vi "AudioTest.SoundCheck Data Log Graph Window - Composite_Smaller.vi"() -> ()   [LabVIEW 2018]
uses:
  TypeDefs/AudioTest.Analysis Data Record.ctl
  TypeDefs/AudioTest.Analysis Folder Navigation Status.ctl
  <vilib>/KATE/Queues/Queue Utils.lvlib
panel:
  in  "Main Tab":enum32{"Data", "Setup"}(tab)
  out "Cmnt":string
  out "Mic Covered Level":string caption="Covered"
  out "Mic Level":string caption="Level"
  out "Right Level":string caption="Level"
  out "Left Level":string caption="Level"
  out "TopEnd":bool
  out "BotEnd":bool
  out "Index":i32
  out "Count":i32
  in  "Folder":path
  out "Loc":string
  in  "MoveFldr":bool
  out "Result":string
  out "Desc":string
  out "Result Code":i32 caption="Code"
  out "Folder":string
  in  "UUTDir Next":bool
  in  "UUTDir Prev":bool
  in  "Snapshot":bool
  out "Name 1 1":string
  out "Graph1 1":cluster{"X":dbl[], "Y":dbl[]}[](graph)
  out "Graph1 2":cluster{"X":dbl[], "Y":dbl[]}[](graph)
  out "Name 1 2":string
  out "Name 3 3":string
  out "Graph3 3":cluster{"X":dbl[], "Y":dbl[]}[](graph)
  out "Name 3 2":string
  out "Graph3 2":cluster{"X":dbl[], "Y":dbl[]}[](graph)
  out "Name 3 1":string
  out "Graph3 1":cluster{"X":dbl[], "Y":dbl[]}[](graph)
  out "Name 2 4":string
  out "Graph2 4":cluster{"X":dbl[], "Y":dbl[]}[](graph)
  out "Graph2 3":cluster{"X":dbl[], "Y":dbl[]}[](graph)
  out "Name 2 3":string
  out "Graph2 2":cluster{"X":dbl[], "Y":dbl[]}[](graph)
  out "Name 2 2":string
  out "Graph2 1":cluster{"X":dbl[], "Y":dbl[]}[](graph)
  out "Name 2 1":string
  out "Graph1 4":cluster{"X":dbl[], "Y":dbl[]}[](graph)
  out "Name 1 4":string
  out "Graph1 3":cluster{"X":dbl[], "Y":dbl[]}[](graph)
  out "Name 1 3":string
  in  "Graphs":T1[](array[typedef])
  in  "QName":string="Plot_Composite"
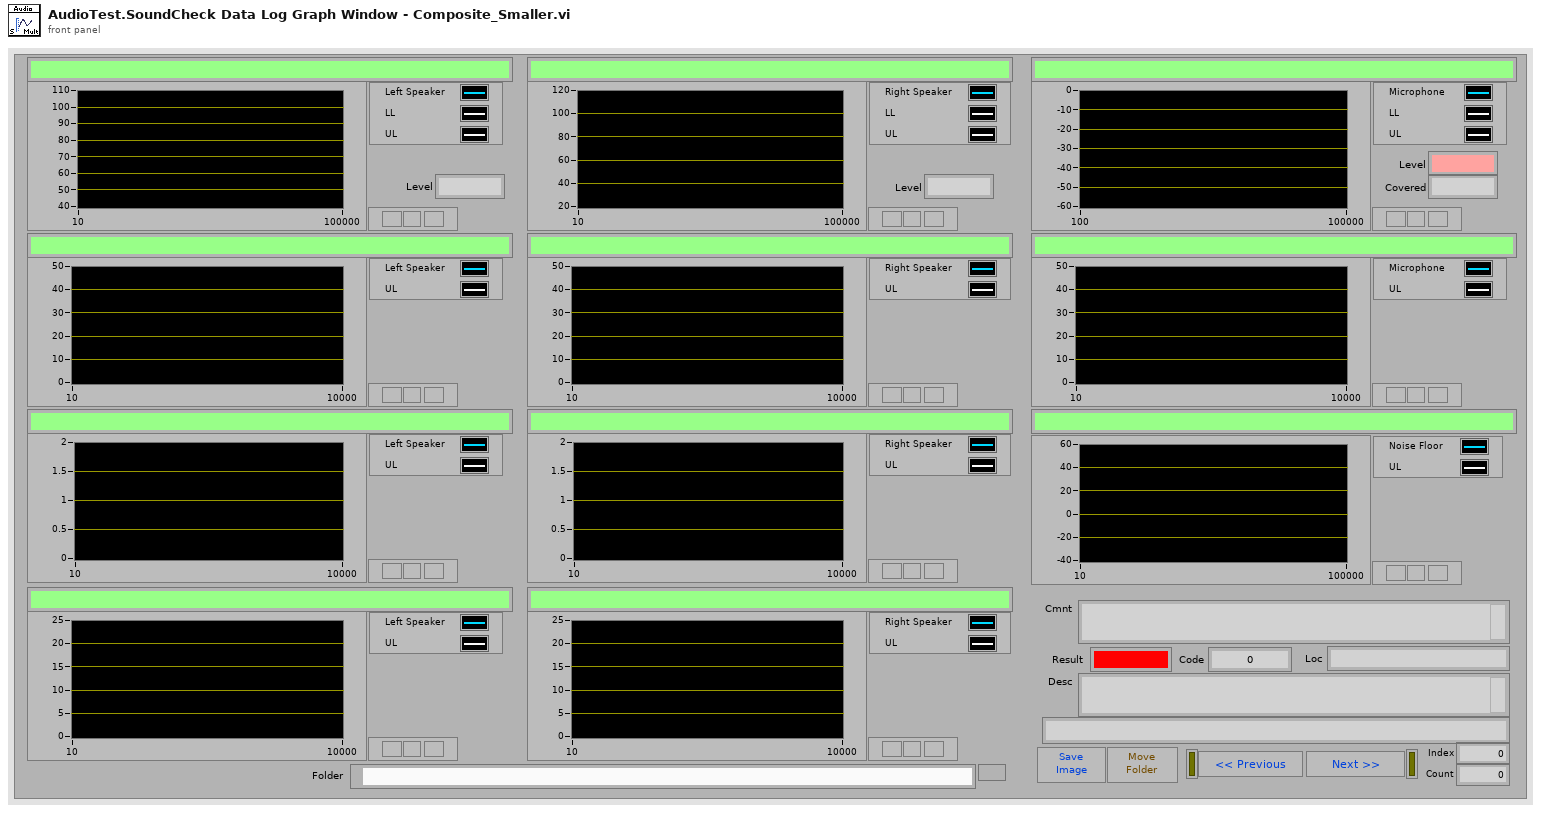
[diagram p1: front panel]
types:
  T1 = typedef "AudioTest.Analysis Data Record.ctl" = cluster{"Name":string, "X Units":string, "Y Units":string, "DataPlots":cluster{"X":dbl[], "Y":dbl[]}[], "LimitPlots":cluster{"X":dbl[], "Y":dbl[]}[], "DataPlotNames":string[], "LimitPlotNames":string[], "Fail":bool}
  T2 = enum32{"Invalid", "Standard", "Closed", "Hidden", "Minimized", "Maximized"}
  T3 = typedef "AudioTest.Analysis Folder Navigation Status.ctl" = cluster{"Index":i32, "Count":i32, "HightEnd":bool, "LowtEnd":bool}
  T4 = cluster{"Graphs":T1[], "PlotColors":u32[], "LimColors":u32[], "Folder":path}
  T5 = typedef "imagedata.ctl" = cluster{"image type":i32, "image depth":i32, "image":u8[], "mask":u8[], "colors":u32[], "Rectangle":cluster{"left":i16, "top":i16, "right":i16, "bottom":i16}}
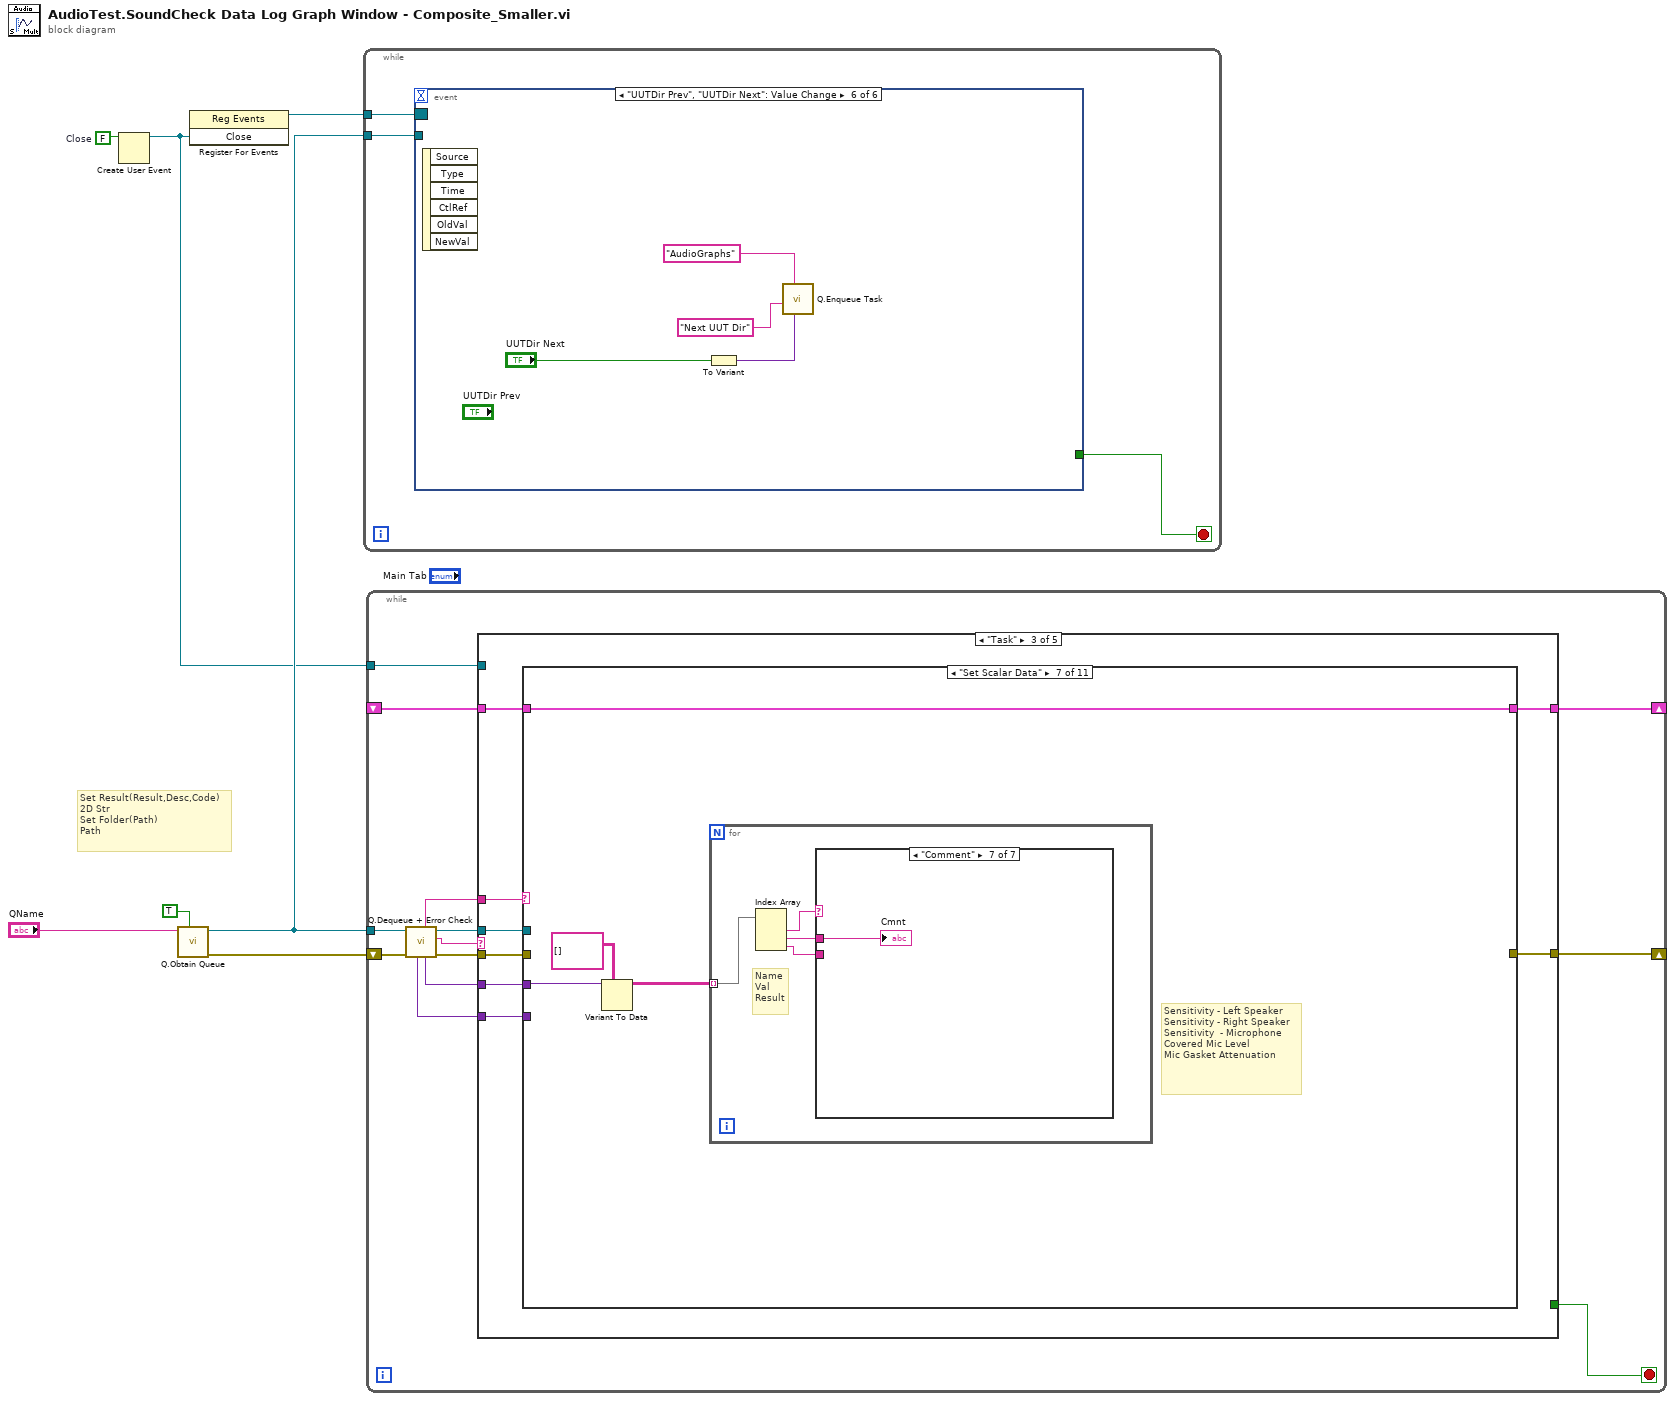
[diagram p0: block diagram]
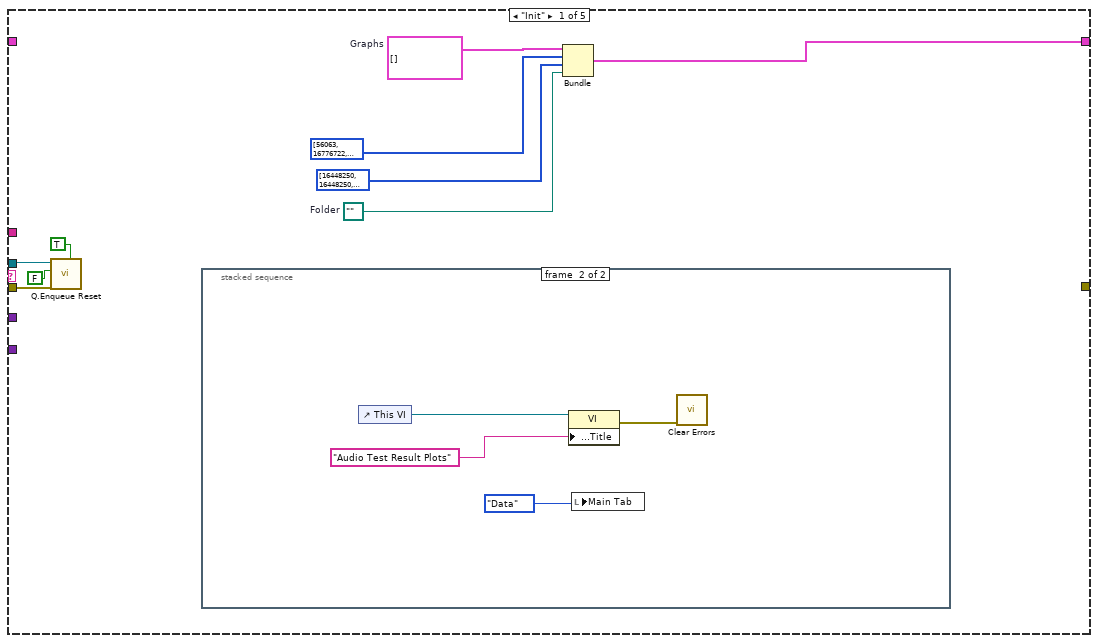
[diagram p2: hidden frame]
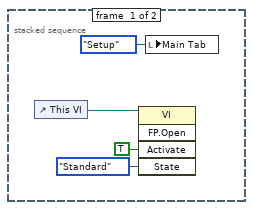
[diagram p3: hidden frame]
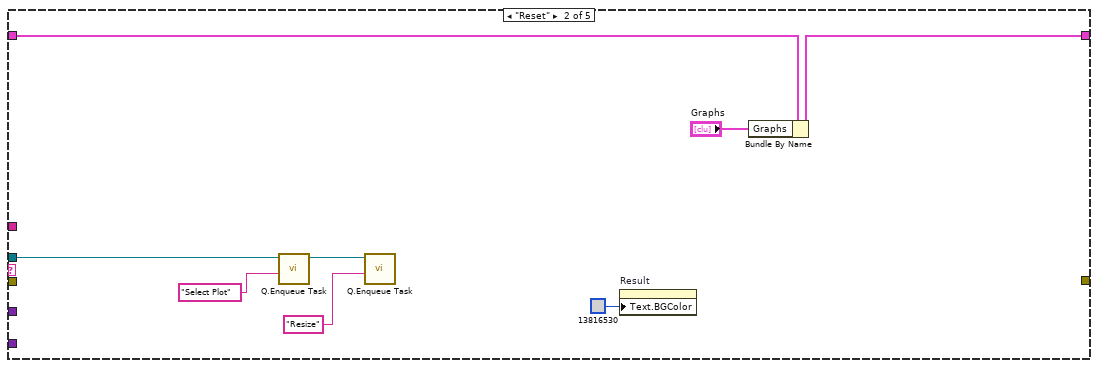
[diagram p4: hidden frame]
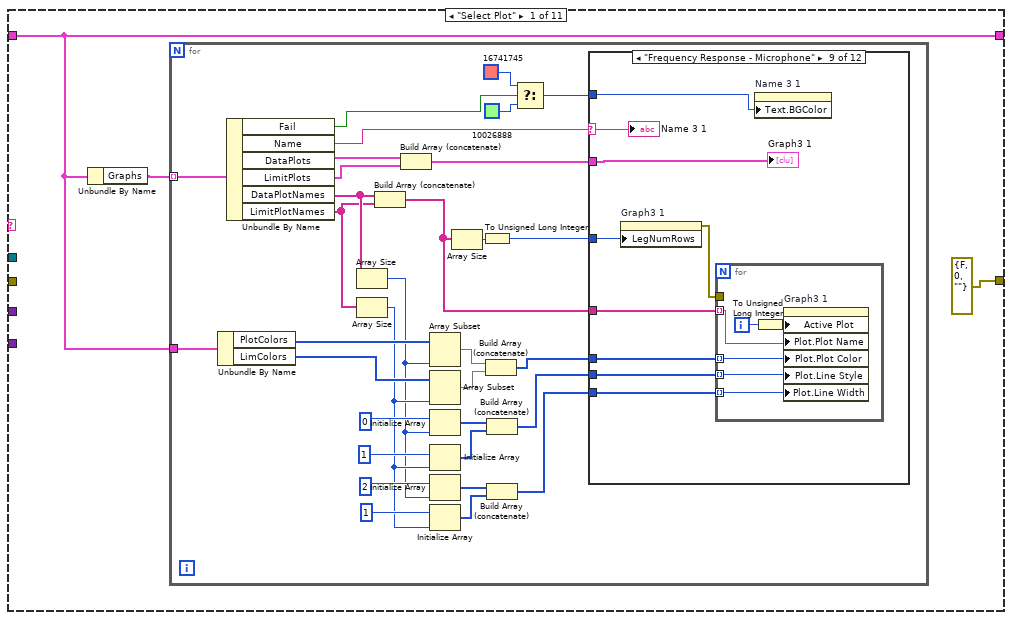
[diagram p5: hidden frame]
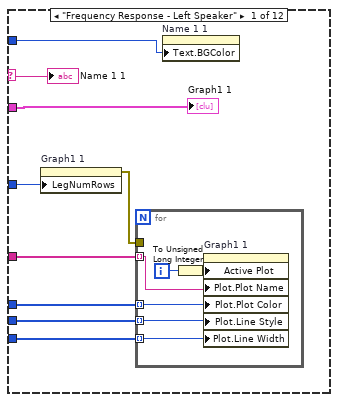
[diagram p6: hidden frame]
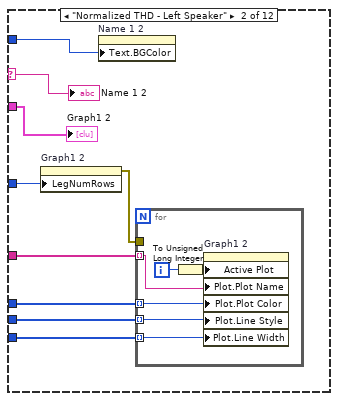
[diagram p7: hidden frame]
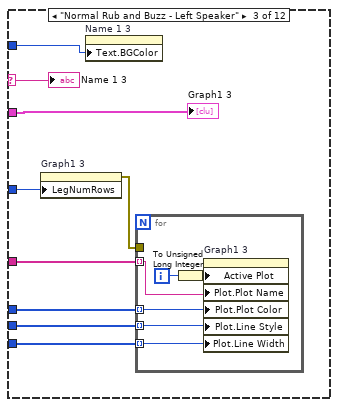
[diagram p8: hidden frame]
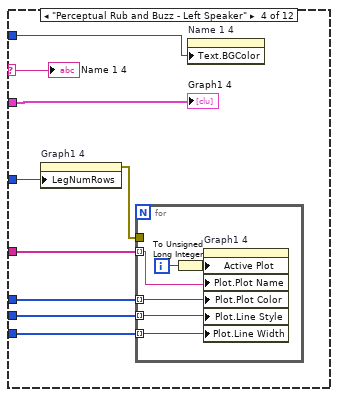
[diagram p9: hidden frame]
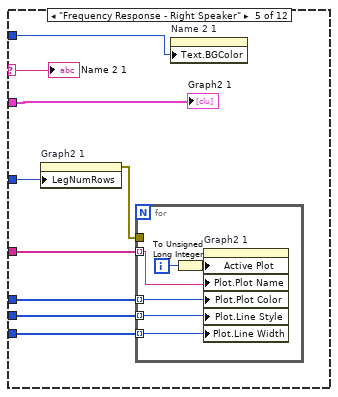
[diagram p10: hidden frame]
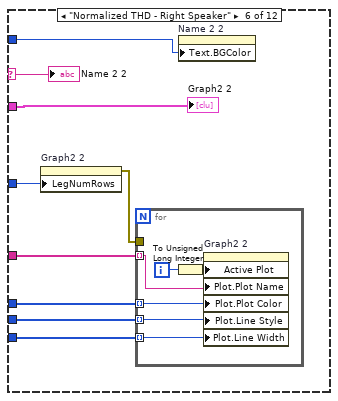
[diagram p11: hidden frame]
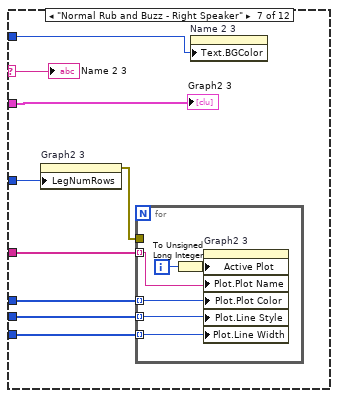
[diagram p12: hidden frame]
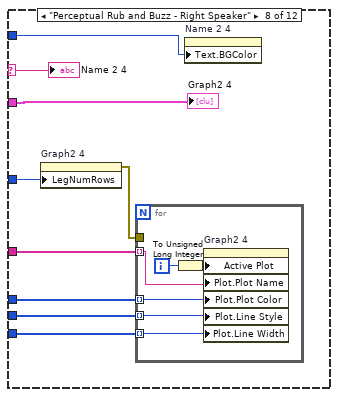
[diagram p13: hidden frame]
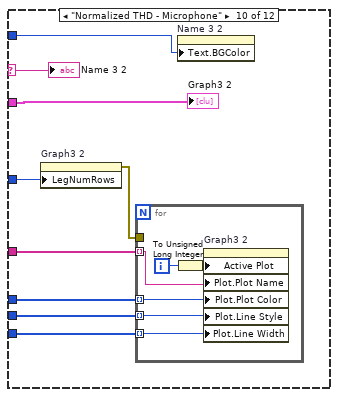
[diagram p14: hidden frame]
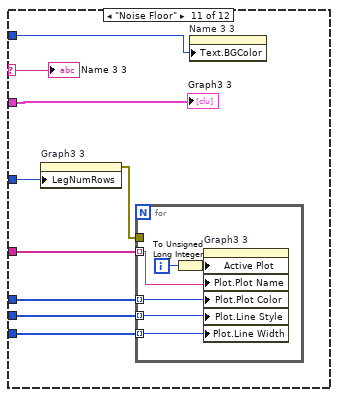
[diagram p15: hidden frame]
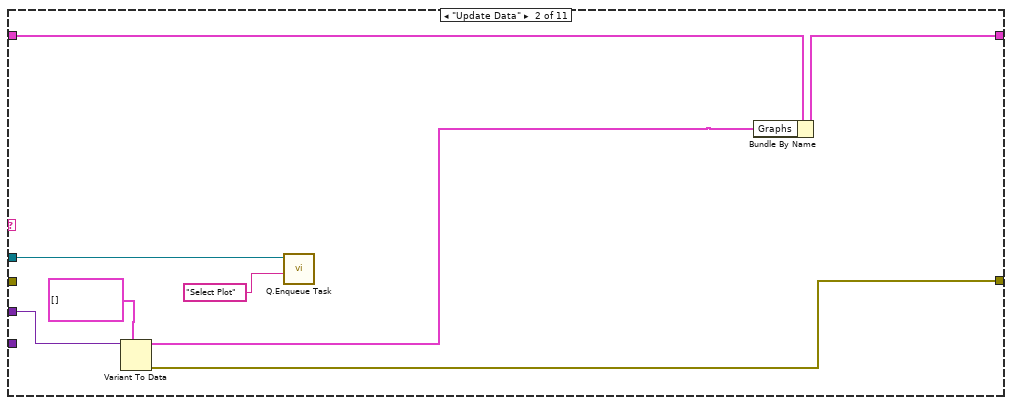
[diagram p17: hidden frame]
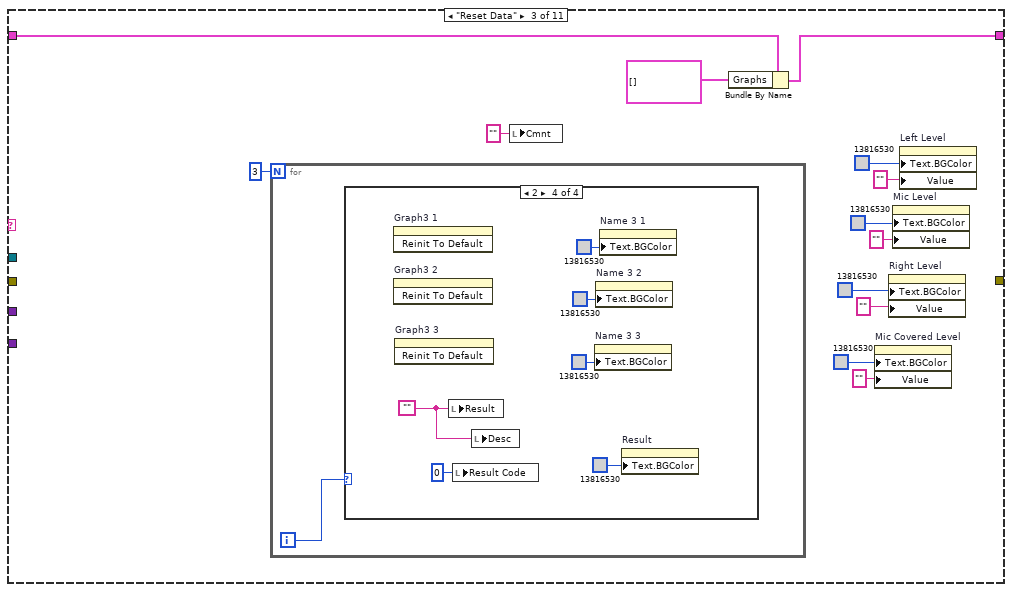
[diagram p18: hidden frame]
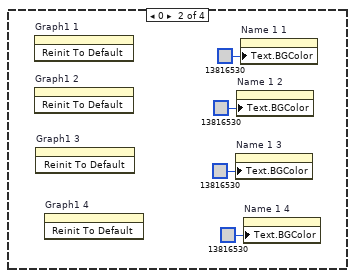
[diagram p20: hidden frame]
diagram:
  w7 = FALSE  # Close
  # "Set Result(Result,Desc,Code)\n2D Str\nSet Folder(Path)\nPath"
  n1 = Create User Event(user event datatype=w7) -> (user event=w2:refnum<user-event>)  [unwired: 1 in, 1 out]
  n2 = call <vilib>:"Q.Obtain Queue.vi"("Enqueue Init"=TRUE, "Q Name"="QName") -> ("error out"=w4:errorcluster, "Q Out"=w3:refnum<queue>)  [unwired: 7 in, 1 out]
  n3 = register-events(w2) -> (reference out=w6:refnum<event-registration>)  [unwired: 2 in, 1 out]
  n4 = while {
    tunnel: w6 -> [w10]
    tunnel: w3 -> [w9]
    stop <- w8 stop-if-true
    n5 = event shown="[5] \"UUTDir Prev\", \"UUTDir Next\": Value Change" {
      selector: w10 -> [_ _ _ _ _ _]
      dyn-events: _ -> [_ _ _ _ _ _]
      timeout: _ -> [_ _ _ _ _ _]
      tunnel: w9 -> [w13 w16 _ w23 w25 _]
      tunnel: [TRUE TRUE _ _ _ _] -> w8
      event Panel Close? {
        n6 = event-data() -> ()  [unwired: 1 in, 4 out]
        n7 = call <vilib>:"Q.Enqueue Exit.vi"("Q In"=w13) -> ("error out"=w12:errorcluster)  [unwired: 9 in, 1 out]
        n8 = call <vilib>:"Clear Errors.vi"("error in (no error)"=w12) -> ()  [unwired: 5 in, 2 out]
        n9 = event-data("Discard?"=TRUE) -> ()  [unwired: 1 in, 1 out]
      }
      event User Event {
        n10 = event-data() -> ()  [unwired: 1 in, 4 out]
        n11 = call <vilib>:"Q.Enqueue Exit.vi"("Q In"=w16) -> ("error out"=w15:errorcluster)  [unwired: 9 in, 1 out]
        n12 = call <vilib>:"Clear Errors.vi"("error in (no error)"=w15) -> ()  [unwired: 5 in, 2 out]
      }
      event "Folder": Value Change {
        n13 = event-data() -> ()  [unwired: 1 in, 6 out]
        n14 = To Variant(anything="Folder") -> (Variant=w21:variant)
        n15 = call <vilib>:"Q.Enqueue Task.vi"("Data1"=w21, "Q Name"="AudioGraphs", "Task Name"="Load Data") -> ()  [unwired: 7 in, 2 out]
      }
      event "Snapshot": Value Change {
        n16 = event-data() -> ()  [unwired: 1 in, 6 out]
        n17 = call <vilib>:"Q.Enqueue Task.vi"("Task Name"="Snapshot", "Q In"=w23) -> ()  [unwired: 8 in, 2 out]
      }
      event "MoveFldr": Value Change {
        n18 = event-data() -> ()  [unwired: 1 in, 6 out]
        n19 = call <vilib>:"Q.Enqueue Task.vi"("Task Name"="MoveFldr", "Q In"=w25) -> ()  [unwired: 8 in, 2 out]
      }
      event "UUTDir Prev", "UUTDir Next": Value Change {
        n20 = event-data() -> ()  [unwired: 1 in, 6 out]
        n21 = To Variant(anything="UUTDir Next") -> (Variant=w27:variant)
        n22 = call <vilib>:"Q.Enqueue Task.vi"("Data1"=w27, "Q Name"="AudioGraphs", "Task Name"="Next UUT Dir") -> ()  [unwired: 7 in, 2 out]
      }
    }
  }
  n23 = while {
    shift-right: [w34] -> _
    shift-left: w4 -> [w39]
    tunnel: w3 -> [w37]
    shift-right: [w32] -> _
    shift-left: _ -> [w31]
    tunnel: w2 -> [w30]
    stop <- w33 stop-if-true
    n24 = call <vilib>:"Q.Dequeue + Error Check.vi"("Error In"=w39, "Q In"=w37) -> ("error out"=w40:errorcluster, "Cmd"=w42:string, "Q Out"=w41:refnum<queue>, "Data1"=w36:variant, "Sub"=w38:string, "Data2"=w35:variant)  [unwired: 4 in]
    n25 = case shown="\"Task\"" w42 {
      tunnel: w41 -> [w51 w65 w74 _ w430]
      tunnel: w40 -> [w50 _ w73 _ _]
      tunnel: w38 -> [_ _ w75 _ _]
      tunnel: w36 -> [_ _ w72 _ _]
      tunnel: w35 -> [_ _ w71 _ _]
      tunnel: [_ _ w68 _ _] -> w34
      tunnel: [_ _ _ _ TRUE] -> w33
      tunnel: [w45 w67 w69 w427 w434] -> w32
      tunnel: w31 -> [_ w66 w70 w428 w434]
      tunnel: w30 -> [_ _ _ _ w433]
      frame "Init" {
        w43 = path ""  # Folder
        w48 = T1[] []  # Graphs
        n26 = call <vilib>:"Q.Enqueue Reset.vi"("Top of Q(T)"=TRUE, "Error In"=w50, "Flush Queue(T)"=FALSE, "Q In"=w51) -> ()  [unwired: 6 in, 2 out]
        n27 = stacked-sequence {
          frame #0 {
            n28 = control-ref of="This VI"() -> (w55:refnum<vi>)
            n29 = invoke class="VI" method="FP.Open"(reference=w55, "Activate"=TRUE ("Activate?"), "State"=T2."Standard") -> ()  [unwired: 2 in, 5 out]
            n30 = local write "Main Tab"(enum32{"Data", "Setup"}."Setup" ("Main Tab")) -> ()
          }
          frame #1 {
            n31 = control-ref of="This VI"() -> (w59:refnum<vi>)
            n32 = property class="VI"(reference=w59, "Front Panel.Title"="Audio Test Result Plots") -> (error out=w58:errorcluster)  [unwired: 1 in, 1 out]
            n33 = local write "Main Tab"(enum32{"Data", "Setup"}."Data" ("Main Tab")) -> ()
            n34 = call <vilib>:"Clear Errors.vi"("error in (no error)"=w58) -> ()  [unwired: 5 in, 2 out]
          }
        }
        n35 = Bundle("Graphs"=w48, "PlotColors"=u32[] [56063, 16776722, 16730898, 16711925, 6618880], "LimColors"=u32[] [16448250, 16448250, 16448250, 16448250, 16448250, 16448250], "Folder"=w43) -> (w45:T4)  [unwired: 1 in]
      }
      frame "Reset" {
        n36 = call <vilib>:"Q.Enqueue Task.vi"("Task Name"="Select Plot", "Q In"=w65) -> ("Q Out"=w62:refnum<queue>)  [unwired: 8 in, 1 out]
        n37 = call <vilib>:"Q.Enqueue Task.vi"("Task Name"="Resize", "Q In"=w62) -> ()  [unwired: 8 in, 2 out]
        n38 = property on="Result" class="Str"("Text.BGColor"=u32 13816530) -> ()  [unwired: 2 in, 2 out]
        n39 = Bundle By Name(cluster=w66, "Graphs"="Graphs") -> (w67:T4)
      }
      frame "Task" {
        n40 = case shown="\"Set Scalar Data\"" w75 {
          tunnel: w74 -> [_ w282 _ _ _ _ _ _ _ _ _]
          tunnel: w73 -> [_ _ _ _ _ _ _ _ _ _ _]
          tunnel: w72 -> [_ w279 _ w314 w323 w334 w342 w378 _ _ _]
          tunnel: w71 -> [_ _ _ _ _ _ _ _ _ _ _]
          tunnel: w70 -> [w78 w281 w295 w317 w325 w335 w343 w371 w387 w407 w424]
          tunnel: [w78 w280 w296 w317 w325 w335 w343 w372 w387 w407 w424] -> w69
          tunnel: [errorcluster {"status"=FALSE, "code"=0, "source"=""} ("error constant") w278 _ _ _ _ _ _ _ _ _] -> w68
          frame "Select Plot" {
            n41 = Unbundle By Name(w78) -> ("Graphs"=w76:T1[])
            n42 = for {
              tunnel: w78 -> [w105]
              tunnel: w76 -> [w84] mode=indexing
              n43 = Unbundle By Name(w105) -> ("PlotColors"=w102:u32[], "LimColors"=w101:u32[])
              n44 = Unbundle By Name(w84) -> ("Fail"=w80:bool, "Name"=w83:string, "DataPlots"=w110:cluster{"X":dbl[], "Y":dbl[]}[], "LimitPlots"=w109:cluster{"X":dbl[], "Y":dbl[]}[], "DataPlotNames"=w104:string[], "LimitPlotNames"=w103:string[])
              n45 = Array Size(array=w104) -> (size(s)=w87:i32)
              n46 = Array Size(array=w103) -> (size(s)=w88:i32)
              n47 = Build Array (concatenate)(w104, w103) -> (w106:string[])
              n48 = Build Array (concatenate)(w110, w109) -> (w85:cluster{"X":dbl[], "Y":dbl[]}[])
              n49 = Array Subset(array=w102, length=w87) -> (w100:u32[])  [unwired: 1 in]
              n50 = Array Subset(array=w101, length=w88) -> (w99:u32[])  [unwired: 1 in]
              n51 = Initialize Array(u8 0 ("Plot.Line Style"), w87) -> (w95:u8[])
              n52 = Initialize Array(u8 1 ("Plot.Line Style"), w88) -> (w94:u8[])
              n53 = Initialize Array(u8 2 ("Plot.Line Style"), w87) -> (w91:u8[])
              n54 = Initialize Array(u8 1 ("Plot.Line Style"), w88) -> (w92:u8[])
              n55 = Array Size(array=w106) -> (size(s)=w108:i32)
              n56 = To Unsigned Long Integer(number=w108) -> (unsigned 32bit integer=w107:u32)
              n57 = Build Array (concatenate)(w100, w99) -> (w98:u32[])
              n58 = Build Array (concatenate)(w95, w94) -> (w93:u8[])
              n59 = Build Array (concatenate)(w91, w92) -> (w86:u8[])
              n60 = Select(t=u32 16741745, s=w80, f=u32 10026888) -> (s? t:f=w79:u32)
              n61 = case shown="\"Frequency Response - Microphone\"" w83 {
                selector: w83 -> [w112 w127 w142 w157 w172 w187 w202 w217 w232 w247 w262 _]
                tunnel: w107 -> [w119 w134 w149 w164 w179 w194 w209 w224 w239 w254 w269 _]
                tunnel: w106 -> [w117 w132 w147 w162 w177 w192 w207 w222 w237 w252 w267 _]
                tunnel: w98 -> [w116 w131 w146 w161 w176 w191 w206 w221 w236 w251 w266 _]
                tunnel: w93 -> [w115 w130 w145 w160 w175 w190 w205 w220 w235 w250 w265 _]
                tunnel: w86 -> [w114 w129 w144 w159 w174 w189 w204 w219 w234 w249 w264 _]
                tunnel: w85 -> [w113 w128 w143 w158 w173 w188 w203 w218 w233 w248 w263 _]
                tunnel: w79 -> [w111 w126 w141 w156 w171 w186 w201 w216 w231 w246 w261 _]
                frame "Frequency Response - Left Speaker" {
                  n62 = property on="Graph1 1" class="XYGraph (strict)"("LegNumRows"=w119) -> (error out=w118:errorcluster)  [unwired: 2 in, 1 out]
                  n63 = for {
                    tunnel: w117 -> [w123] mode=indexing
                    tunnel: w118 -> [_]
                    tunnel: w116 -> [w122] mode=indexing
                    tunnel: w115 -> [w121] mode=indexing
                    tunnel: w114 -> [w120] mode=indexing
                    i -> [w124]
                    n64 = To Unsigned Long Integer(number=w124) -> (unsigned 32bit integer=w125:u32)
                    n65 = property on="Graph1 1" class="XYGraph (strict)"("Active Plot"=w125, "Plot.Plot Name"=w123, "Plot.Plot Color"=w122, "Plot.Line Style"=w121, "Plot.Line Width"=w120) -> ()  [unwired: 2 in, 2 out]
                  }
                  n66 = property on="Name 1 1" class="Str"("Text.BGColor"=w111) -> ()  [unwired: 2 in, 2 out]
                  "Graph1 1" <- w113
                  "Name 1 1" <- w112
                }
                frame "Normalized THD - Left Speaker" {
                  n67 = property on="Graph1 2" class="XYGraph (strict)"("LegNumRows"=w134) -> (error out=w133:errorcluster)  [unwired: 2 in, 1 out]
                  n68 = property on="Name 1 2" class="Str"("Text.BGColor"=w126) -> ()  [unwired: 2 in, 2 out]
                  n69 = for {
                    tunnel: w132 -> [w138] mode=indexing
                    tunnel: w133 -> [_]
                    tunnel: w131 -> [w137] mode=indexing
                    tunnel: w130 -> [w136] mode=indexing
                    tunnel: w129 -> [w135] mode=indexing
                    i -> [w139]
                    n70 = To Unsigned Long Integer(number=w139) -> (unsigned 32bit integer=w140:u32)
                    n71 = property on="Graph1 2" class="XYGraph (strict)"("Active Plot"=w140, "Plot.Plot Name"=w138, "Plot.Plot Color"=w137, "Plot.Line Style"=w136, "Plot.Line Width"=w135) -> ()  [unwired: 2 in, 2 out]
                  }
                  "Graph1 2" <- w128
                  "Name 1 2" <- w127
                }
                frame "Normal Rub and Buzz - Left Speaker" {
                  n72 = property on="Graph1 3" class="XYGraph (strict)"("LegNumRows"=w149) -> (error out=w148:errorcluster)  [unwired: 2 in, 1 out]
                  n73 = property on="Name 1 3" class="Str"("Text.BGColor"=w141) -> ()  [unwired: 2 in, 2 out]
                  n74 = for {
                    tunnel: w147 -> [w153] mode=indexing
                    tunnel: w148 -> [_]
                    tunnel: w146 -> [w152] mode=indexing
                    tunnel: w145 -> [w151] mode=indexing
                    tunnel: w144 -> [w150] mode=indexing
                    i -> [w154]
                    n75 = To Unsigned Long Integer(number=w154) -> (unsigned 32bit integer=w155:u32)
                    n76 = property on="Graph1 3" class="XYGraph (strict)"("Active Plot"=w155, "Plot.Plot Name"=w153, "Plot.Plot Color"=w152, "Plot.Line Style"=w151, "Plot.Line Width"=w150) -> ()  [unwired: 2 in, 2 out]
                  }
                  "Graph1 3" <- w143
                  "Name 1 3" <- w142
                }
                frame "Perceptual Rub and Buzz - Left Speaker" {
                  n77 = property on="Graph1 4" class="XYGraph (strict)"("LegNumRows"=w164) -> (error out=w163:errorcluster)  [unwired: 2 in, 1 out]
                  n78 = for {
                    tunnel: w162 -> [w168] mode=indexing
                    tunnel: w163 -> [_]
                    tunnel: w161 -> [w167] mode=indexing
                    tunnel: w160 -> [w166] mode=indexing
                    tunnel: w159 -> [w165] mode=indexing
                    i -> [w169]
                    n79 = To Unsigned Long Integer(number=w169) -> (unsigned 32bit integer=w170:u32)
                    n80 = property on="Graph1 4" class="XYGraph (strict)"("Active Plot"=w170, "Plot.Plot Name"=w168, "Plot.Plot Color"=w167, "Plot.Line Style"=w166, "Plot.Line Width"=w165) -> ()  [unwired: 2 in, 2 out]
                  }
                  n81 = property on="Name 1 4" class="Str"("Text.BGColor"=w156) -> ()  [unwired: 2 in, 2 out]
                  "Graph1 4" <- w158
                  "Name 1 4" <- w157
                }
                frame "Frequency Response - Right Speaker" {
                  n82 = property on="Graph2 1" class="XYGraph (strict)"("LegNumRows"=w179) -> (error out=w178:errorcluster)  [unwired: 2 in, 1 out]
                  n83 = for {
                    tunnel: w177 -> [w183] mode=indexing
                    tunnel: w178 -> [_]
                    tunnel: w176 -> [w182] mode=indexing
                    tunnel: w175 -> [w181] mode=indexing
                    tunnel: w174 -> [w180] mode=indexing
                    i -> [w184]
                    n84 = To Unsigned Long Integer(number=w184) -> (unsigned 32bit integer=w185:u32)
                    n85 = property on="Graph2 1" class="XYGraph (strict)"("Active Plot"=w185, "Plot.Plot Name"=w183, "Plot.Plot Color"=w182, "Plot.Line Style"=w181, "Plot.Line Width"=w180) -> ()  [unwired: 2 in, 2 out]
                  }
                  n86 = property on="Name 2 1" class="Str"("Text.BGColor"=w171) -> ()  [unwired: 2 in, 2 out]
                  "Graph2 1" <- w173
                  "Name 2 1" <- w172
                }
                frame "Normalized THD - Right Speaker" {
                  n87 = property on="Graph2 2" class="XYGraph (strict)"("LegNumRows"=w194) -> (error out=w193:errorcluster)  [unwired: 2 in, 1 out]
                  n88 = for {
                    tunnel: w192 -> [w198] mode=indexing
                    tunnel: w193 -> [_]
                    tunnel: w191 -> [w197] mode=indexing
                    tunnel: w190 -> [w196] mode=indexing
                    tunnel: w189 -> [w195] mode=indexing
                    i -> [w199]
                    n89 = To Unsigned Long Integer(number=w199) -> (unsigned 32bit integer=w200:u32)
                    n90 = property on="Graph2 2" class="XYGraph (strict)"("Active Plot"=w200, "Plot.Plot Name"=w198, "Plot.Plot Color"=w197, "Plot.Line Style"=w196, "Plot.Line Width"=w195) -> ()  [unwired: 2 in, 2 out]
                  }
                  n91 = property on="Name 2 2" class="Str"("Text.BGColor"=w186) -> ()  [unwired: 2 in, 2 out]
                  "Graph2 2" <- w188
                  "Name 2 2" <- w187
                }
                frame "Normal Rub and Buzz - Right Speaker" {
                  n92 = property on="Graph2 3" class="XYGraph (strict)"("LegNumRows"=w209) -> (error out=w208:errorcluster)  [unwired: 2 in, 1 out]
                  n93 = for {
                    tunnel: w207 -> [w213] mode=indexing
                    tunnel: w208 -> [_]
                    tunnel: w206 -> [w212] mode=indexing
                    tunnel: w205 -> [w211] mode=indexing
                    tunnel: w204 -> [w210] mode=indexing
                    i -> [w214]
                    n94 = To Unsigned Long Integer(number=w214) -> (unsigned 32bit integer=w215:u32)
                    n95 = property on="Graph2 3" class="XYGraph (strict)"("Active Plot"=w215, "Plot.Plot Name"=w213, "Plot.Plot Color"=w212, "Plot.Line Style"=w211, "Plot.Line Width"=w210) -> ()  [unwired: 2 in, 2 out]
                  }
                  n96 = property on="Name 2 3" class="Str"("Text.BGColor"=w201) -> ()  [unwired: 2 in, 2 out]
                  "Graph2 3" <- w203
                  "Name 2 3" <- w202
                }
                frame "Perceptual Rub and Buzz - Right Speaker" {
                  n97 = property on="Graph2 4" class="XYGraph (strict)"("LegNumRows"=w224) -> (error out=w223:errorcluster)  [unwired: 2 in, 1 out]
                  n98 = for {
                    tunnel: w222 -> [w228] mode=indexing
                    tunnel: w223 -> [_]
                    tunnel: w221 -> [w227] mode=indexing
                    tunnel: w220 -> [w226] mode=indexing
                    tunnel: w219 -> [w225] mode=indexing
                    i -> [w229]
                    n99 = To Unsigned Long Integer(number=w229) -> (unsigned 32bit integer=w230:u32)
                    n100 = property on="Graph2 4" class="XYGraph (strict)"("Active Plot"=w230, "Plot.Plot Name"=w228, "Plot.Plot Color"=w227, "Plot.Line Style"=w226, "Plot.Line Width"=w225) -> ()  [unwired: 2 in, 2 out]
                  }
                  n101 = property on="Name 2 4" class="Str"("Text.BGColor"=w216) -> ()  [unwired: 2 in, 2 out]
                  "Graph2 4" <- w218
                  "Name 2 4" <- w217
                }
                frame "Frequency Response - Microphone" {
                  n102 = property on="Graph3 1" class="XYGraph (strict)"("LegNumRows"=w239) -> (error out=w238:errorcluster)  [unwired: 2 in, 1 out]
                  n103 = for {
                    tunnel: w237 -> [w243] mode=indexing
                    tunnel: w238 -> [_]
                    tunnel: w236 -> [w242] mode=indexing
                    tunnel: w235 -> [w241] mode=indexing
                    tunnel: w234 -> [w240] mode=indexing
                    i -> [w244]
                    n104 = To Unsigned Long Integer(number=w244) -> (unsigned 32bit integer=w245:u32)
                    n105 = property on="Graph3 1" class="XYGraph (strict)"("Active Plot"=w245, "Plot.Plot Name"=w243, "Plot.Plot Color"=w242, "Plot.Line Style"=w241, "Plot.Line Width"=w240) -> ()  [unwired: 2 in, 2 out]
                  }
                  n106 = property on="Name 3 1" class="Str"("Text.BGColor"=w231) -> ()  [unwired: 2 in, 2 out]
                  "Graph3 1" <- w233
                  "Name 3 1" <- w232
                }
                frame "Normalized THD - Microphone" {
                  n107 = property on="Graph3 2" class="XYGraph (strict)"("LegNumRows"=w254) -> (error out=w253:errorcluster)  [unwired: 2 in, 1 out]
                  n108 = for {
                    tunnel: w252 -> [w258] mode=indexing
                    tunnel: w253 -> [_]
                    tunnel: w251 -> [w257] mode=indexing
                    tunnel: w250 -> [w256] mode=indexing
                    tunnel: w249 -> [w255] mode=indexing
                    i -> [w259]
                    n109 = To Unsigned Long Integer(number=w259) -> (unsigned 32bit integer=w260:u32)
                    n110 = property on="Graph3 2" class="XYGraph (strict)"("Active Plot"=w260, "Plot.Plot Name"=w258, "Plot.Plot Color"=w257, "Plot.Line Style"=w256, "Plot.Line Width"=w255) -> ()  [unwired: 2 in, 2 out]
                  }
                  n111 = property on="Name 3 2" class="Str"("Text.BGColor"=w246) -> ()  [unwired: 2 in, 2 out]
                  "Graph3 2" <- w248
                  "Name 3 2" <- w247
                }
                frame "Noise Floor" {
                  n112 = property on="Graph3 3" class="XYGraph (strict)"("LegNumRows"=w269) -> (error out=w268:errorcluster)  [unwired: 2 in, 1 out]
                  n113 = for {
                    tunnel: w267 -> [w273] mode=indexing
                    tunnel: w268 -> [_]
                    tunnel: w266 -> [w272] mode=indexing
                    tunnel: w265 -> [w271] mode=indexing
                    tunnel: w264 -> [w270] mode=indexing
                    i -> [w274]
                    n114 = To Unsigned Long Integer(number=w274) -> (unsigned 32bit integer=w275:u32)
                    n115 = property on="Graph3 3" class="XYGraph (strict)"("Active Plot"=w275, "Plot.Plot Name"=w273, "Plot.Plot Color"=w272, "Plot.Line Style"=w271, "Plot.Line Width"=w270) -> ()  [unwired: 2 in, 2 out]
                  }
                  n116 = property on="Name 3 3" class="Str"("Text.BGColor"=w261) -> ()  [unwired: 2 in, 2 out]
                  "Graph3 3" <- w263
                  "Name 3 3" <- w262
                }
                frame Default {
                }
              }
            }
          }
          frame "Update Data" {
            n117 = Variant To Data(type=T1[] [] ("Graphs"), Variant=w279) -> (data=w277:T1[], error out=w278:errorcluster)  [unwired: 1 in]
            n118 = call <vilib>:"Q.Enqueue Task.vi"("Task Name"="Select Plot", "Q In"=w282) -> ()  [unwired: 8 in, 2 out]
            n119 = Bundle By Name(cluster=w281, "Graphs"=w277) -> (w280:T4)
          }
          frame "Reset Data" {
            n120 = for {
              N: 3 -> [_]
              i -> [w297]
              n121 = case shown="2" w297 {
                frame Default {
                }
                frame 0 {
                  n122 = invoke on="Graph1 1" class="XYGraph (strict)" method="Reinit To Default"() -> ()  [unwired: 3 in, 3 out]
                  n123 = invoke on="Graph1 2" class="XYGraph (strict)" method="Reinit To Default"() -> ()  [unwired: 3 in, 3 out]
                  n124 = invoke on="Graph1 3" class="XYGraph (strict)" method="Reinit To Default"() -> ()  [unwired: 3 in, 3 out]
                  n125 = invoke on="Graph1 4" class="XYGraph (strict)" method="Reinit To Default"() -> ()  [unwired: 3 in, 3 out]
                  n126 = property on="Name 1 3" class="Str"("Text.BGColor"=u32 13816530) -> ()  [unwired: 2 in, 2 out]
                  n127 = property on="Name 1 2" class="Str"("Text.BGColor"=u32 13816530) -> ()  [unwired: 2 in, 2 out]
                  n128 = property on="Name 1 1" class="Str"("Text.BGColor"=u32 13816530) -> ()  [unwired: 2 in, 2 out]
                  n129 = property on="Name 1 4" class="Str"("Text.BGColor"=u32 13816530) -> ()  [unwired: 2 in, 2 out]
                }
                frame 1 {
                  n130 = invoke on="Graph2 1" class="XYGraph (strict)" method="Reinit To Default"() -> ()  [unwired: 3 in, 3 out]
                  n131 = invoke on="Graph2 2" class="XYGraph (strict)" method="Reinit To Default"() -> ()  [unwired: 3 in, 3 out]
                  n132 = invoke on="Graph2 3" class="XYGraph (strict)" method="Reinit To Default"() -> ()  [unwired: 3 in, 3 out]
                  n133 = invoke on="Graph2 4" class="XYGraph (strict)" method="Reinit To Default"() -> ()  [unwired: 3 in, 3 out]
                  n134 = property on="Name 2 3" class="Str"("Text.BGColor"=u32 13816530) -> ()  [unwired: 2 in, 2 out]
                  n135 = property on="Name 2 2" class="Str"("Text.BGColor"=u32 13816530) -> ()  [unwired: 2 in, 2 out]
                  n136 = property on="Name 2 1" class="Str"("Text.BGColor"=u32 13816530) -> ()  [unwired: 2 in, 2 out]
                  n137 = property on="Name 2 4" class="Str"("Text.BGColor"=u32 13816530) -> ()  [unwired: 2 in, 2 out]
                }
                frame 2 {
                  w308 = ""
                  n138 = invoke on="Graph3 1" class="XYGraph (strict)" method="Reinit To Default"() -> ()  [unwired: 3 in, 3 out]
                  n139 = invoke on="Graph3 2" class="XYGraph (strict)" method="Reinit To Default"() -> ()  [unwired: 3 in, 3 out]
                  n140 = invoke on="Graph3 3" class="XYGraph (strict)" method="Reinit To Default"() -> ()  [unwired: 3 in, 3 out]
                  n141 = local write "Result"(w308) -> ()
                  n142 = local write "Result Code"(0 ("Result Code")) -> ()
                  n143 = local write "Desc"(w308) -> ()
                  n144 = property on="Name 3 3" class="Str"("Text.BGColor"=u32 13816530) -> ()  [unwired: 2 in, 2 out]
                  n145 = property on="Name 3 2" class="Str"("Text.BGColor"=u32 13816530) -> ()  [unwired: 2 in, 2 out]
                  n146 = property on="Name 3 1" class="Str"("Text.BGColor"=u32 13816530) -> ()  [unwired: 2 in, 2 out]
                  n147 = property on="Result" class="Str"("Text.BGColor"=u32 13816530) -> ()  [unwired: 2 in, 2 out]
                }
              }
            }
            n148 = local write "Cmnt"("" ("Cmnt")) -> ()
            n149 = Bundle By Name(cluster=w295, "Graphs"=T1[] []) -> (w296:T4)
            n150 = property on="Mic Covered Level" class="Str"("Text.BGColor"=u32 13816530, "Value"="" ("Mic Level")) -> ()  [unwired: 2 in, 2 out]
            n151 = property on="Right Level" class="Str"("Text.BGColor"=u32 13816530, "Value"="" ("Mic Level")) -> ()  [unwired: 2 in, 2 out]
            n152 = property on="Mic Level" class="Str"("Text.BGColor"=u32 13816530, "Value"="" ("Mic Level")) -> ()  [unwired: 2 in, 2 out]
            n153 = property on="Left Level" class="Str"("Text.BGColor"=u32 13816530, "Value"="" ("Mic Level")) -> ()  [unwired: 2 in, 2 out]
          }
          frame "Set Title" {
            n154 = Variant To Data(type="", Variant=w314) -> (data=w312:string)  [unwired: 1 in, 1 out]
            n155 = control-ref of="This VI"() -> (w316:refnum<vi>)
            n156 = property class="VI"(reference=w316, "Front Panel.Title"=w312) -> (error out=w315:errorcluster)  [unwired: 1 in, 1 out]
            n157 = call <vilib>:"Clear Errors.vi"("error in (no error)"=w315) -> ()  [unwired: 5 in, 2 out]
          }
          frame "DirNav" {
            n158 = Variant To Data(type=T3 {"Index"=0, "Count"=0, "HightEnd"=FALSE, "LowtEnd"=FALSE} ("FolderNavStatus"), Variant=w323) -> (data=w318:T3)  [unwired: 1 in, 1 out]
            n159 = Unbundle By Name(w318) -> ("Index"=→"Index":i32, "Count"=→"Count":i32, "HightEnd"=→"TopEnd":bool, "LowtEnd"=→"BotEnd":bool)
          }
          frame "Set Result" {
            n160 = Variant To Data(type=string[] [], Variant=w334) -> (data=w332:string[])  [unwired: 1 in, 1 out]
            n161 = Index Array(array=w332) -> (element #1=w326:string, element #2=w330:string, element #3=→"Desc":string, element #4=→"Loc":string)  [unwired: 4 in]
            "Result" <- w326
            n162 = Decimal String To Number(string=w330) -> (number=→"Result Code":i32)  [unwired: 2 in, 1 out]
            n163 = case shown="\"Error\"" w326 {
              tunnel: [u32 6618880 u32 16711680 u32 16758290 u32 13816530] -> w327
              frame "Pass" {
              }
              frame "Fail" {
              }
              frame "Error" {
              }
              frame Default {
              }
            }
            n164 = property on="Result" class="Str"("Text.BGColor"=w327) -> ()  [unwired: 2 in, 2 out]
          }
          frame "Set Scalar Data" {
            # "Sensitivity - Left Speaker\nSensitivity - Right Speaker\nSensitivity  - Microphone\nCovered Mic Level\nMic Gasket Attenuation"
            n165 = Variant To Data(type=string[][] [], Variant=w342) -> (data=w340:string[][])  [unwired: 1 in, 1 out]
            n166 = for {
              tunnel: w340 -> [w347] mode=indexing
              # "Name\nVal\nResult"
              n167 = Index Array(array=w347) -> (element #1=w346:string, element #2=w345:string, element #3=w344:string)  [unwired: 3 in]
              n168 = case shown="\"Comment\"" w346 {
                tunnel: w345 -> [_ w348 w353 w358 w363 _ w368]
                tunnel: w344 -> [_ w350 w355 w360 _ w365 _]
                frame "False", Default {
                }
                frame "Sensitivity - Left Speaker" {
                  n169 = case shown="\"FAIL\"" w350 {
                    tunnel: [u32 13816530 u32 16753568] -> w349
                    frame Default {
                    }
                    frame "FAIL" {
                    }
                  }
                  n170 = property on="Left Level" class="Str"("Text.BGColor"=w349) -> ()  [unwired: 2 in, 2 out]
                  "Left Level" <- w348
                }
                frame "Sensitivity - Right Speaker" {
                  n171 = case shown="\"FAIL\"" w355 {
                    tunnel: [u32 13816530 u32 16753568] -> w354
                    frame Default {
                    }
                    frame "FAIL" {
                    }
                  }
                  n172 = property on="Right Level" class="Str"("Text.BGColor"=w354) -> ()  [unwired: 2 in, 2 out]
                  "Right Level" <- w353
                }
                frame "Sensitivity  - Microphone" {
                  n173 = case shown="Default" w360 {
                    tunnel: [u32 13816530 u32 16753568] -> w359
                    frame Default {
                    }
                    frame "FAIL" {
                    }
                  }
                  n174 = property on="Mic Level" class="Str"("Text.BGColor"=w359) -> ()  [unwired: 2 in, 2 out]
                  "Mic Level" <- w358
                }
                frame "Covered Mic Level" {
                  "Mic Covered Level" <- w363
                }
                frame "Mic Gasket Attenuation" {
                  n175 = case shown="\"FAIL\"" w365 {
                    tunnel: [u32 13816530 u32 16753568] -> w364
                    frame Default {
                    }
                    frame "FAIL" {
                    }
                  }
                  n176 = property on="Mic Covered Level" class="Str"("Text.BGColor"=w364) -> ()  [unwired: 2 in, 2 out]
                }
                frame "Comment" {
                  "Cmnt" <- w368
                }
              }
            }
          }
          frame "Set Folder" {
            n177 = Variant To Data(type=path "", Variant=w378) -> (data=w370:path)  [unwired: 1 in, 1 out]
            n178 = File/Directory Info(path=w370) -> (path out=w375:path, directory=w376:bool, error out=w369:errorcluster)  [unwired: 1 in, 4 out]
            n179 = Bundle By Name(cluster=w371, "Folder"=w370) -> (w372:T4)
            n180 = local write "Folder"(w370) -> ()
            n181 = case shown="False" w376 {
              tunnel: w375 -> [w379 w381]
              tunnel: [w380 w381] -> w374
              tunnel: w369 -> [_ _]
              frame False {
                n182 = Strip Path(path=w379) -> (stripped path=w380:path)  [unwired: 1 out]
              }
              frame True {
              }
            }
            n183 = Strip Path(path=w374) -> (name=→"Folder":string)  [unwired: 1 out]
          }
          frame "Snapshot" {
            n184 = Unbundle By Name(w387) -> ("Folder"=w386:path)
            n185 = local read "Folder"() -> (w384:string)
            n186 = Format Into String(format string="%s_AudioGraphs.png" ("default name"), w384) -> (resulting string=w383:string)  [unwired: 2 in, 1 out]
            n187 = control-ref of="This VI"() -> (w392:refnum<vi>)
            n188 = invoke class="VI" method="FP.Get Image"(reference=w392, "visible area only"=FALSE ("Visible Area Only"), "image depth"=24 ("Image Depth")) -> ("image data"=w393:T5)  [unwired: 3 in, 5 out]
            n189 = call "File Dialog"("start path"=w386, "prompt"="Select path to save screen shot", "default name"=w383, "pattern (all files)"="*.png") -> ("selected path"=w394:path, "cancelled"=w395:bool, "error out"=w382:errorcluster)  [unwired: 8 in, 1 out]
            n190 = case shown="No Error" w382 {
              tunnel: w395 -> [w398 _]
              tunnel: w394 -> [w397 _]
              tunnel: w393 -> [w396 _]
              frame No Error {
                n191 = case shown="False" w398 {
                  tunnel: w396 -> [w401 _]
                  tunnel: [w400 _] -> _
                  tunnel: w397 -> [w399 _]
                  frame False {
                    n192 = call <vilib>:"Write PNG File.vi"("image data"=w401, "path to PNG file"=w399) -> ("error out"=w400:errorcluster)  [unwired: 8 in, 1 out]
                  }
                  frame True {
                  }
                }
              }
              frame Error {
              }
            }
          }
          frame "MoveFldr" {
            n193 = Unbundle By Name(w407) -> ("Folder"=w403:path)
            n194 = Strip Path(path=w403) -> (stripped path=w404:path, name=w406:string)
            n195 = call "File Dialog2"("start path"=w404, "prompt"="Move Folder to New Location.", "default name"=w406) -> ("selected path"=w408:path, "cancelled"=w409:bool, "error out"=w402:errorcluster)  [unwired: 9 in, 1 out]
            n196 = case shown="No Error" w402 {
              tunnel: w409 -> [w412 _]
              tunnel: w408 -> [w411 _]
              tunnel: w403 -> [w410 _]
              frame No Error {
                n197 = case shown="False" w412 {
                  tunnel: w411 -> [w415 _]
                  tunnel: w410 -> [w414 _]
                  tunnel: [w413 _] -> _
                  frame False {
                    n198 = stacked-sequence {
                      tunnel: w415 -> [_ _ w423]
                      tunnel: w414 -> [_ _ w422]
                      tunnel: [_ _ w421] -> w413
                      frame #0 {
                        n199 = To Variant(anything=TRUE) -> (Variant=w419:variant)
                        n200 = call <vilib>:"Q.Enqueue Task.vi"("Data1"=w419, "Q Name"="AudioGraphs", "Task Name"="Next UUT Dir") -> ()  [unwired: 7 in, 2 out]
                      }
                      frame #1 {
                        n201 = Wait (ms)(milliseconds to wait=u32 200) -> ()  [unwired: 1 out]
                      }
                      frame #2 {
                        n202 = Move(source path=w422, 10:w423) -> (error out=w421:errorcluster)  [unwired: 3 in, 2 out]
                      }
                    }
                  }
                  frame True {
                  }
                }
              }
              frame Error {
              }
            }
          }
          frame Default {
          }
        }
      }
      frame "Error", Default {
        # "Do Nothing (for now)"
        n203 = local write "Graph1 1"(cluster{"X":dbl[], "Y":dbl[]}[] [] ("XY Graph")) -> ()
        n204 = Bundle By Name(cluster=w428, "Graphs"=T1[] []) -> (w427:T4)
      }
      frame "Exit" {
        n205 = Release Queue(queue=w430, force destroy? (F)=TRUE) -> ()  [unwired: 1 in, 3 out]
        n206 = Generate User Event(user event=w433, event data cluster=TRUE ("event data")) -> ()  [unwired: 2 in, 2 out]
        n207 = case shown="True" TRUE {
          tunnel: [_ w436] -> _
          frame False {
          }
          frame True {
            n208 = control-ref of="This VI"() -> (w438:refnum<vi>)
            n209 = invoke class="VI" method="FP.Close"(reference=w438) -> (error out=w437:errorcluster)  [unwired: 2 in, 2 out]
            n210 = Close Reference(reference=w438, error in (no error)=w437) -> (error out=w436:errorcluster)
          }
        }
      }
    }
  }
